vi "set Draw Triangles.vi"(10 "Draw Triangles":bool, 11 "Scene in":refnum<class "Scene.lvclass">) -> (3 "Scene out":refnum<class "Scene.lvclass">)   [LabVIEW 2020, in "Scene.lvclass"]
uses:
  Scene.lvclass
  Scene.lvclass/Scene.ctl
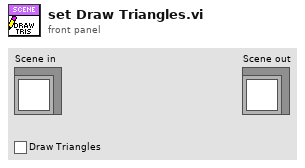
[diagram p1: front panel]
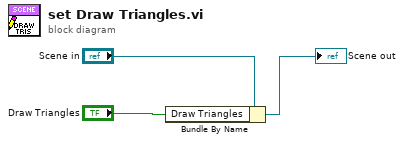
[diagram p0: block diagram]
diagram:
  n1 = Bundle By Name(cluster="Scene in", "Draw Triangles"="Draw Triangles") -> (→"Scene out":refnum<class "Scene.lvclass">)
